vi "AddTestSuite_WithParent_TagNameIncludesParentTag.vi"() -> (0 "error out":errorcluster)   [LabVIEW 2019, in "ResultTreeTest.lvlib"]
uses:
  ResultTreeTest.lvlib
  2a6c7ef5-d8ea-4de4-ba7d-c6663dbf2225.vi
  Constraint/IsEqual/Create.vi
  Constraint/IsEqual/IsEqual.lvclass
  ResultTree/ResultTree.lvclass
panel:
  in  "Tree":string(tree)
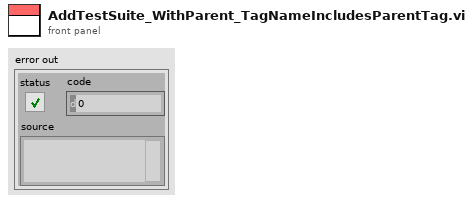
[diagram p1: front panel]
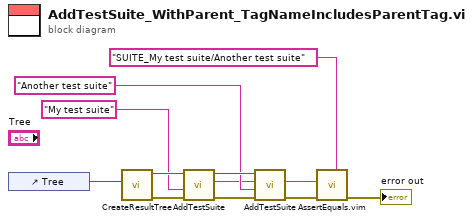
[diagram p0: block diagram]
diagram:
  n1 = control-ref of="Tree"() -> (w11:refnum<vi>)
  n2 = call "CreateResultTree.vi"("Tree Refnum"=w11) -> ("error out"=w10:errorcluster, "ResultTree out"=w9:refnum<class "ResultTree.lvclass">)  [unwired: 9 in]
  n3 = call "AddTestSuite.vi"("error in (no error)"=w10, "Name"="My test suite", "ResultTree in"=w9) -> ("error out"=w6:errorcluster, "Tag Name"=w3:string, "ResultTree out"=w7:refnum<class "ResultTree.lvclass">)  [unwired: 6 in]
  n4 = call "AddTestSuite.vi"("error in (no error)"=w6, "Name"="Another test suite", "Parent Tag (\"\")"=w3, "ResultTree in"=w7) -> ("error out"=w1:errorcluster, "Tag Name"=w2:string)  [unwired: 5 in, 1 out]
  n5 = call "AssertEquals.vim"("Expected"="SUITE_My test suite/Another test suite" ("Name"), "error in (no error)"=w1, "Actual"=w2) -> ("error out"=→"error out":errorcluster)  [unwired: 8 in]
